vi "Get Field Names.vi"(10 "Fields":T1[](array[typedef])) -> (2 "Field Names":string[](array[string]))   [LabVIEW 2014, in "hse-db.lvlib" / "MySQL (TCP).lvlib"]
uses:
  MySQL (TCP).lvlib
  Controls/Fields.ctl
  Controls/Character Set.ctl
  Controls/Data Types.ctl
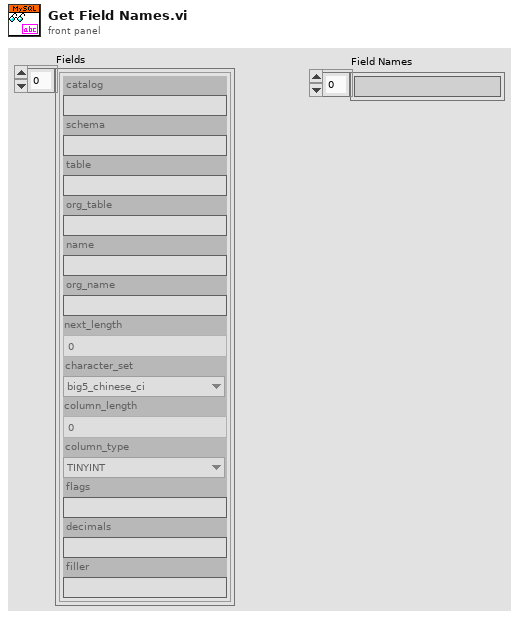
[diagram p1: front panel]
types:
  T1 = typedef "hse-db.lvlib/MySQL (TCP).lvlib/Fields.ctl" = cluster{"catalog":string, "schema":string, "table":string, "org_table":string, "name":string, "org_name":string, "next_length":u64, "character_set":T2, "column_length":u64, "column_type":T3, "flags":string, "decimals":string, "filler":string}
  T2 = typedef "hse-db.lvlib/MySQL (TCP).lvlib/Character Set.ctl" = enum16{"big5_chinese_ci", "dec8_swedish_ci", "cp850_general_ci", "hp8_english_ci", "koi8r_general_ci", "latin1_swedish_ci", "latin2_general_ci", "swe7_swedish_ci", "ascii_general_ci", "ujis_japanese_ci", "sjis_japanese_ci", "hebrew_general_ci", "tis620_thai_ci", "euckr_korean_ci", "koi8u_general_ci", "gb2312_chinese_ci", "greek_general_ci", "cp1250_general_ci", "gbk_chinese_ci", "latin5_turkish_ci", "armscii8_general_ci", "utf8_general_ci", "ucs2_general_ci", "cp866_general_ci", "keybcs2_general_ci", "macce_general_ci", "macroman_general_ci", "cp852_general_ci", "latin7_general_ci", "cp1251_general_ci", "utf16_general_ci", "utf16le_general_ci", "cp1256_general_ci", "cp1257_general_ci", "utf32_general_ci", "binary", "geostd8_general_ci", "cp932_japanese_ci", "eucjpms_japanese_ci", "gb18030_chinese_ci", "utf8mb4_0900_ai_ci"}
  T3 = typedef "hse-db.lvlib/MySQL (TCP).lvlib/Data Types.ctl" = enum16{"TINYINT", "SMALLINT", "MEDIUMINT", "INT", "BIGINT", "FLOAT", "DOUBLE", "NULL", "DECIMAL", "BIT", "CHAR", "VARCHAR", "TINYTEXT", "TEXT", "MEDIUMTEXT", "LONGTEXT", "BINARY", "VARBINARY", "TINYBLOB", "BLOB", "MEDIUMBLOB", "LONGBLOB", "ENUM", "SET", "DATE", "DATETIME", "TIME", "TIMESTAMP", "YEAR", "GEOMETRY"}
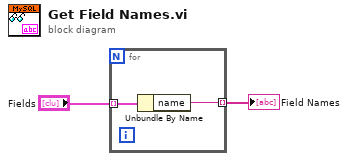
[diagram p0: block diagram]
diagram:
  n1 = for {
    tunnel: "Fields" -> [w4] mode=indexing
    tunnel: [w3] -> w1 mode=indexing
    n2 = Unbundle By Name(w4) -> ("name"=w3:string)
  }
  "Field Names" <- w1
